vi "Close SV.vi"(8 "error in (no error)":errorcluster, 10 "Process Name":string="Flow Module 1", 11 "State Cluster in":T1={"Settings"={"Feed Module Configuration"={"Cycle Period"=0.0, "Ismatech"={"VISA resource name"="", "Simulated?"=FALSE, "Pump Number"=1.0, "Reverse?"=FALSE}, "Masterflex"={"VISA resource name"="", "Simulated?"=FALSE, "Pump Number"=1.0, "Reverse?"=FALSE}, "Mettler"={"VISA resource name"="", "Simulated?"=FALSE}, "Bronkhorst M13 Flow Meter"={"VISA resource name"="", "Simulated?"=FALSE, "Smoothing Steps"=1}, "PID 2 Parameters"={"Input Device"=enum."Flowmeter", "Output Device"=enum."Ismatec ISM 831C", "Setpoint"=0.0, "PID gains"={"proportional gain (Kc)"=1.0, "integral time (Ti, min)"=0.01, "derivative time (Td, min)"=0.0}}, "Manual Entry"=0.0, "Auto?"=TRUE, "VICI Settings"={"VISA resource name"="", "Simulated?"=FALSE, "Pump Number"=0.0, "Reverse?"=FALSE}, "output range"={"output high"=100.0, "output low"=0.0}}, "Load Count"=0.0, "TT Configuration In"={"physical channels"="cDAQ2Mod4/ai0", "name to assign"="Temp1", "units"=10143}, "PT Configuration"={"physical channels"="cDAQ2Mod8/ai15", "name to assign"="Pressure", "units"=10342}}, "Shared Variables"={"PID 1 Process Variable"="PID1-Mettler Toledo Scale 1", "PID 1 Output"="PID1-Mettler Toledo Scale 1", "PID 1 Setpoint"="PID1-Setpoint", "PID 1 Setpoint SV refnum"="ni.var.psp://localhost/Flow Module 1/PID1-Setpoint", "PID 1 Process Variable SV refnum"="ni.var.psp://localhost/Flow Module 1/PID1-Setpoint", "PID 1 Output SV refnum"="ni.var.psp://localhost/Flow Module 1/PID1-Setpoint"}, "Feed Module Config"={"GUID"="", "Drop Coords"={"Horizontal"=0, "Vertical"=0}, "Process Name"="", "Settings"={"Cycle Period"=500.0, "Ismatech"={"VISA resource name"="", "Simulated?"=TRUE, "Pump Number"=1.0, "Reverse?"=FALSE}, "Masterflex"={"VISA resource name"="", "Simulated?"=TRUE, "Pump Number"=1.0, "Reverse?"=FALSE}, "Mettler"={"VISA resource name"="", "Simulated?"=FALSE}, "Bronkhorst M13 Flow Meter"={"VISA resource name"="", "Simulated?"=TRUE, "Smoothing Steps"=1}, "PID 2 Parameters"={"Input Device"=enum."Default", "Output Device"=enum."Default", "Setpoint"=0.0, "PID gains"={"proportional gain (Kc)"=1.0, "integral time (Ti, min)"=0.01, "derivative time (Td, min)"=0.0}}, "Manual Entry"=0.0, "Auto?"=TRUE, "VICI Settings"={"VISA resource name"="", "Simulated?"=TRUE, "Pump Number"=0.0, "Reverse?"=FALSE}, "output range"={"output high"=100.0, "output low"=0.0}}, "Load Count"=0}} {"Feed Module Config"."Settings"."output range"."output low" min=0.0 max=100.0 format="%.2f"; "Feed Module Config"."Settings"."output range"."output high" format="%.2f"; "Feed Module Config"."Settings"."VICI Settings"."Pump Number" min=1.0 max=20.0 step=1.0; "Feed Module Config"."Settings"."PID 2 Parameters"."PID gains"."derivative time (Td, min)" format="%.3f"; "Feed Module Config"."Settings"."PID 2 Parameters"."PID gains"."integral time (Ti, min)" format="%.3f"; "Feed Module Config"."Settings"."PID 2 Parameters"."PID gains"."proportional gain (Kc)" format="%.3f"; "Feed Module Config"."Settings"."Bronkhorst M13 Flow Meter"."Smoothing Steps" min=1 step=1; "Feed Module Config"."Settings"."Masterflex"."Pump Number" min=1.0 max=20.0 step=1.0; "Feed Module Config"."Settings"."Ismatech"."Pump Number" min=1.0 max=20.0 step=1.0; "Settings"."PT Configuration"."units" items=["Amps"=10342, "From Custom Scale"=10065]; "Settings"."TT Configuration In"."units" items=["Deg C"=10143, "Deg F"=10144, "Kelvins"=10325, "Deg R"=10145, "From Custom Scale"=10065]; "Settings"."Feed Module Configuration"."output range"."output low" min=0.0 max=100.0 format="%.2f"; "Settings"."Feed Module Configuration"."output range"."output high" format="%.2f"; "Settings"."Feed Module Configuration"."VICI Settings"."Pump Number" min=1.0 max=20.0 step=1.0; "Settings"."Feed Module Configuration"."PID 2 Parameters"."PID gains"."derivative time (Td, min)" format="%.3f"; "Settings"."Feed Module Configuration"."PID 2 Parameters"."PID gains"."integral time (Ti, min)" format="%.3f"; "Settings"."Feed Module Configuration"."PID 2 Parameters"."PID gains"."proportional gain (Kc)" format="%.3f"; "Settings"."Feed Module Configuration"."Bronkhorst M13 Flow Meter"."Smoothing Steps" min=1 step=1; "Settings"."Feed Module Configuration"."Masterflex"."Pump Number" min=1.0 max=20.0 step=1.0; "Settings"."Feed Module Configuration"."Ismatech"."Pump Number" min=1.0 max=20.0 step=1.0}) -> (0 "error out":errorcluster, 3 "State Cluster out":T1={"Settings"={"Feed Module Configuration"={"Cycle Period"=0.0, "Ismatech"={"VISA resource name"="", "Simulated?"=FALSE, "Pump Number"=1.0, "Reverse?"=FALSE}, "Masterflex"={"VISA resource name"="", "Simulated?"=FALSE, "Pump Number"=1.0, "Reverse?"=FALSE}, "Mettler"={"VISA resource name"="", "Simulated?"=FALSE}, "Bronkhorst M13 Flow Meter"={"VISA resource name"="", "Simulated?"=FALSE, "Smoothing Steps"=1}, "PID 2 Parameters"={"Input Device"=enum."Flowmeter", "Output Device"=enum."Ismatec ISM 831C", "Setpoint"=0.0, "PID gains"={"proportional gain (Kc)"=1.0, "integral time (Ti, min)"=0.01, "derivative time (Td, min)"=0.0}}, "Manual Entry"=0.0, "Auto?"=TRUE, "VICI Settings"={"VISA resource name"="", "Simulated?"=FALSE, "Pump Number"=0.0, "Reverse?"=FALSE}, "output range"={"output high"=100.0, "output low"=0.0}}, "Load Count"=0.0, "TT Configuration In"={"physical channels"="cDAQ2Mod4/ai0", "name to assign"="Temp1", "units"=10143}, "PT Configuration"={"physical channels"="cDAQ2Mod8/ai15", "name to assign"="Pressure", "units"=10342}}, "Shared Variables"={"PID 1 Process Variable"="PID1-Mettler Toledo Scale 1", "PID 1 Output"="PID1-Mettler Toledo Scale 1", "PID 1 Setpoint"="PID1-Setpoint", "PID 1 Setpoint SV refnum"="ni.var.psp://localhost/Flow Module 1/PID1-Setpoint", "PID 1 Process Variable SV refnum"="ni.var.psp://localhost/Flow Module 1/PID1-Setpoint", "PID 1 Output SV refnum"="ni.var.psp://localhost/Flow Module 1/PID1-Setpoint"}, "Feed Module Config"={"GUID"="", "Drop Coords"={"Horizontal"=0, "Vertical"=0}, "Process Name"="", "Settings"={"Cycle Period"=500.0, "Ismatech"={"VISA resource name"="", "Simulated?"=TRUE, "Pump Number"=1.0, "Reverse?"=FALSE}, "Masterflex"={"VISA resource name"="", "Simulated?"=TRUE, "Pump Number"=1.0, "Reverse?"=FALSE}, "Mettler"={"VISA resource name"="", "Simulated?"=FALSE}, "Bronkhorst M13 Flow Meter"={"VISA resource name"="", "Simulated?"=TRUE, "Smoothing Steps"=1}, "PID 2 Parameters"={"Input Device"=enum."Default", "Output Device"=enum."Default", "Setpoint"=0.0, "PID gains"={"proportional gain (Kc)"=1.0, "integral time (Ti, min)"=0.01, "derivative time (Td, min)"=0.0}}, "Manual Entry"=0.0, "Auto?"=TRUE, "VICI Settings"={"VISA resource name"="", "Simulated?"=TRUE, "Pump Number"=0.0, "Reverse?"=FALSE}, "output range"={"output high"=100.0, "output low"=0.0}}, "Load Count"=0}} {"Feed Module Config"."Settings"."output range"."output low" min=0.0 max=100.0 format="%.2f"; "Feed Module Config"."Settings"."output range"."output high" format="%.2f"; "Feed Module Config"."Settings"."VICI Settings"."Pump Number" min=1.0 max=20.0 step=1.0; "Feed Module Config"."Settings"."PID 2 Parameters"."PID gains"."derivative time (Td, min)" format="%.3f"; "Feed Module Config"."Settings"."PID 2 Parameters"."PID gains"."integral time (Ti, min)" format="%.3f"; "Feed Module Config"."Settings"."PID 2 Parameters"."PID gains"."proportional gain (Kc)" format="%.3f"; "Feed Module Config"."Settings"."Bronkhorst M13 Flow Meter"."Smoothing Steps" min=1 step=1; "Feed Module Config"."Settings"."Masterflex"."Pump Number" min=1.0 max=20.0 step=1.0; "Feed Module Config"."Settings"."Ismatech"."Pump Number" min=1.0 max=20.0 step=1.0; "Settings"."PT Configuration"."units" items=["Amps"=10342, "From Custom Scale"=10065]; "Settings"."TT Configuration In"."units" items=["Deg C"=10143, "Deg F"=10144, "Kelvins"=10325, "Deg R"=10145, "From Custom Scale"=10065]; "Settings"."Feed Module Configuration"."output range"."output low" min=0.0 max=100.0 format="%.2f"; "Settings"."Feed Module Configuration"."output range"."output high" format="%.2f"; "Settings"."Feed Module Configuration"."VICI Settings"."Pump Number" min=1.0 max=20.0 step=1.0; "Settings"."Feed Module Configuration"."PID 2 Parameters"."PID gains"."derivative time (Td, min)" format="%.3f"; "Settings"."Feed Module Configuration"."PID 2 Parameters"."PID gains"."integral time (Ti, min)" format="%.3f"; "Settings"."Feed Module Configuration"."PID 2 Parameters"."PID gains"."proportional gain (Kc)" format="%.3f"; "Settings"."Feed Module Configuration"."Bronkhorst M13 Flow Meter"."Smoothing Steps" min=1 step=1; "Settings"."Feed Module Configuration"."Masterflex"."Pump Number" min=1.0 max=20.0 step=1.0; "Settings"."Feed Module Configuration"."Ismatech"."Pump Number" min=1.0 max=20.0 step=1.0})   [LabVIEW 2021, in "Scale Module.lvlib"]
uses:
  Scale Module.lvlib
  Shared Variables/Dynamic Shared Variables.lvlib
  Controls/Scale Module Shared Variable Cluster.ctl
  Controls/Scale Module Settings Cluster.ctl
  Settings/Settings.ctl
  Settings/Settings.lvlib
  Controls/Scale Module State Cluster.ctl
  Ismatec ISM 831C/Controls/Ismatech Settings Cluster.ctl
  Masterflex 7550-30/Controls/Settings Cluster.ctl
  Masterflex 7550-30/Masterflex 7550-30.lvlib
  Mettler Toledo/Controls/Settings Cluster.ctl
  Mettler Toledo/Mettler Toledo.lvlib
  Bronkhorst M13 Flow Meter/Settings Cluster.ctl
  Bronkhorst M13 Flow Meter/Bronkhorst M13 Flow Meter.lvlib
  Measure Instrument/PID Input Enum.ctl
  Measure Instrument/PID 2 Output Enum.ctl
  Measure Instrument/PID 2 Parameters Cluster.ctl
  Pressure Sensor/PT Configuration.ctl
  Pressure Sensor/Pressure.lvlib
  VICI M50/VICI Settings.ctl
  <vilib>/Utility/miscctls.llb/LVPoint32TypeDef.ctl
  Controls/Scale Module Config Cluster.ctl
panel:
  # "Output Instruments"
  # "Input Instruments"
  # "Output Instruments"
  # "Input Instruments"
  # "Output Instruments"
  # "Input Instruments"
  # "Output Instruments"
  # "Input Instruments"
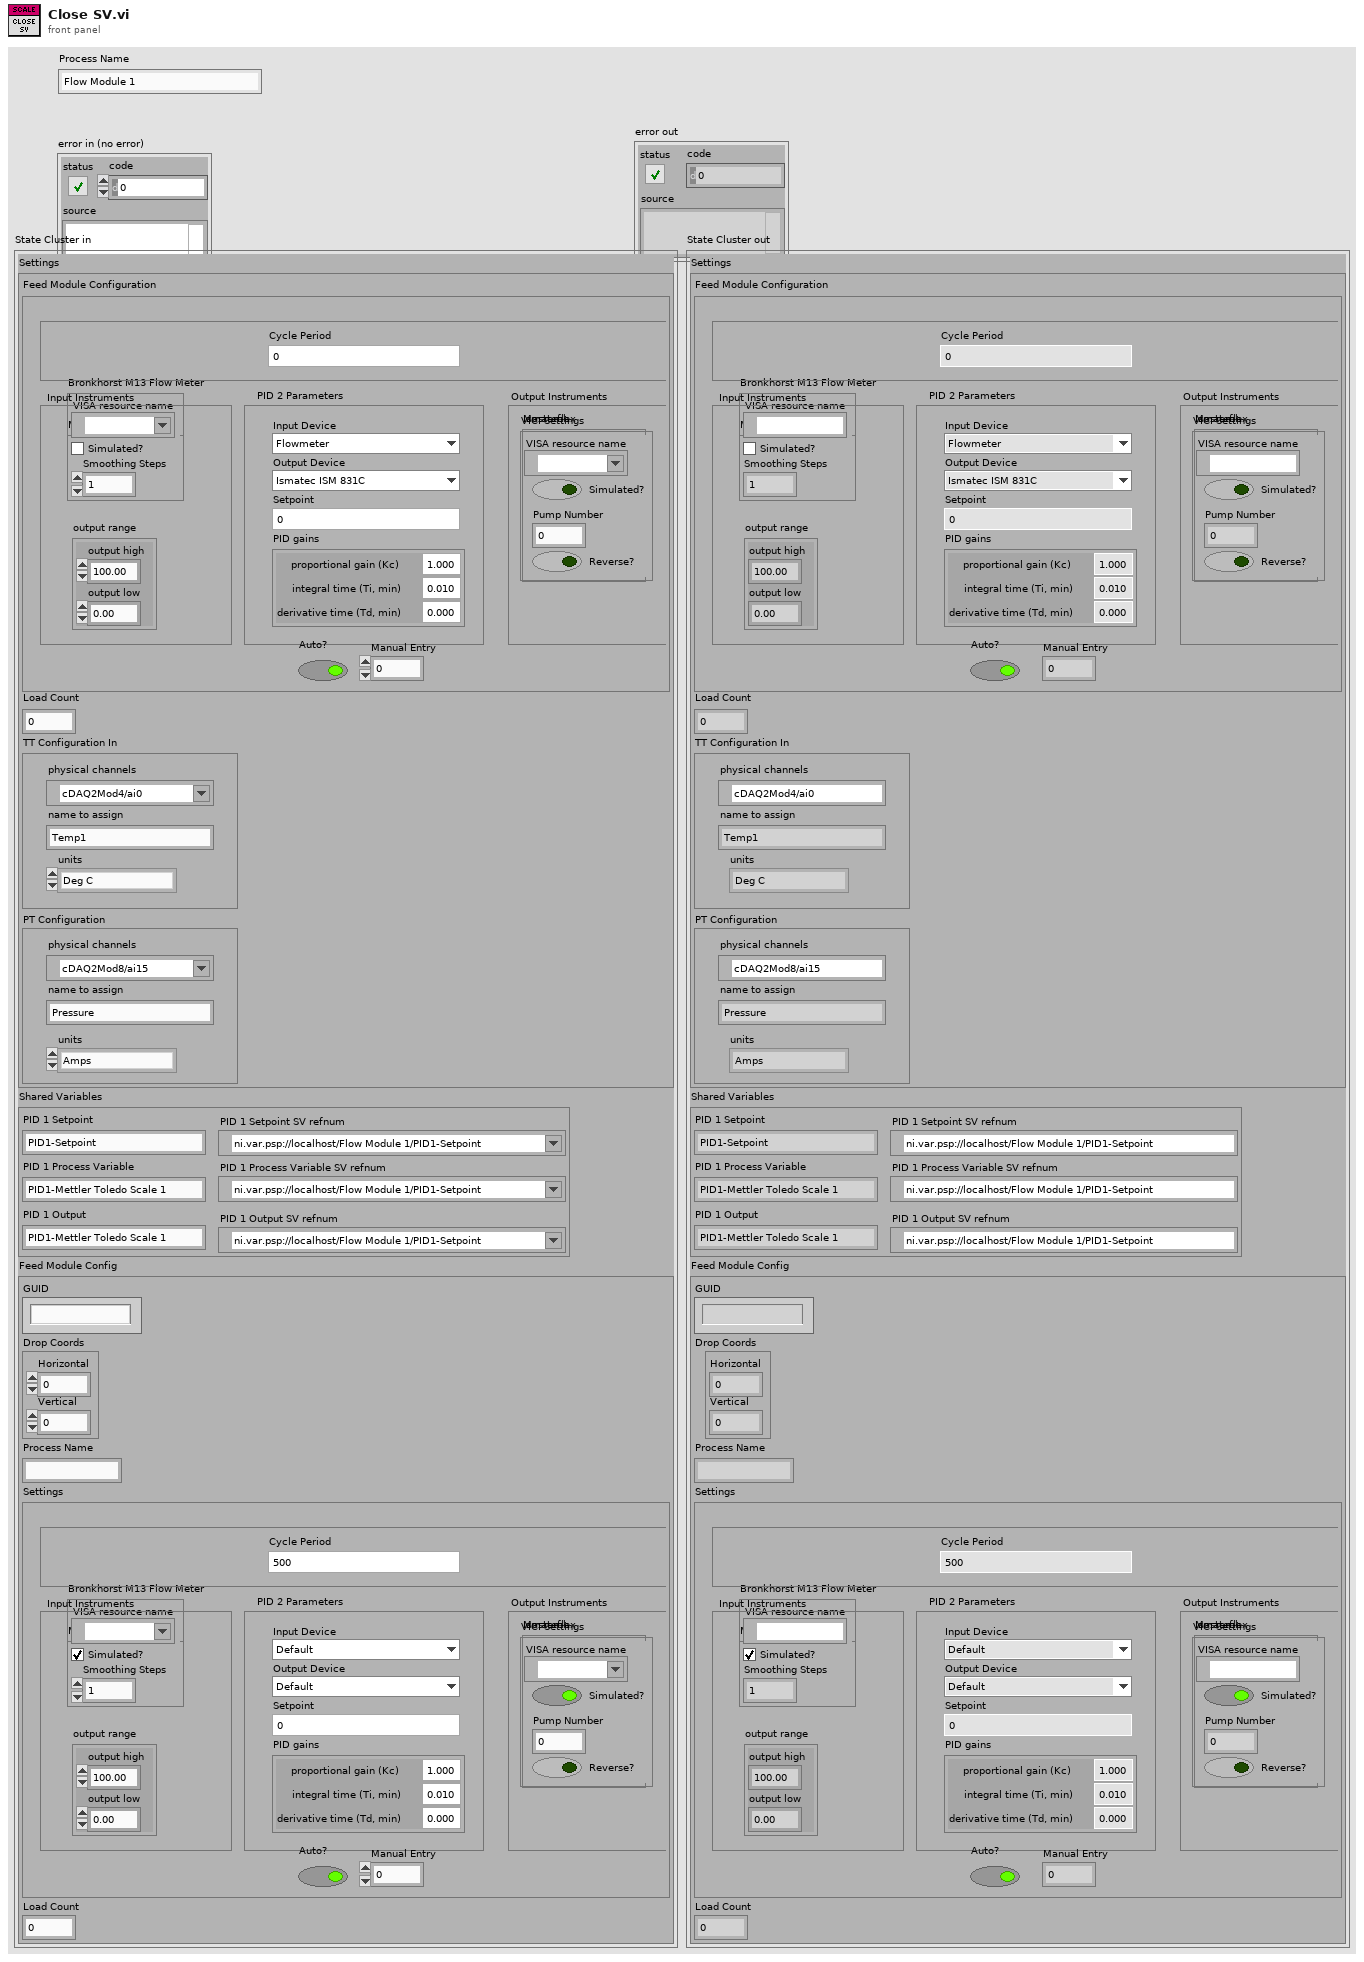
[diagram p1: front panel]
types:
  T1 = typedef "Scale Module.lvlib/Scale Module State Cluster.ctl" = cluster{"Settings":T2, "Shared Variables":T13, "Feed Module Config":T14}
  T2 = typedef "Settings.lvlib/Settings.ctl" = cluster{"Feed Module Configuration":T3, "Load Count":dbl, "TT Configuration In":cluster{"physical channels":tag, "name to assign":string, "units":i32}, "PT Configuration":T12}
  T3 = typedef "Scale Module.lvlib/Scale Module Settings Cluster.ctl" = cluster{"Cycle Period":dbl, "Ismatech":T4, "Masterflex":T5, "Mettler":T6, "Bronkhorst M13 Flow Meter":T7, "PID 2 Parameters":T8, "Manual Entry":dbl, "Auto?":bool, "VICI Settings":T11, "output range":cluster{"output high":dbl, "output low":dbl}}
  T4 = typedef "Ismatec ISM 831C.lvlib/Ismatech Settings Cluster.ctl" = cluster{"VISA resource name":refnum<visa-resource-name>, "Simulated?":bool, "Pump Number":dbl, "Reverse?":bool}
  T5 = typedef "Masterflex 7550-30.lvlib/Settings Cluster.ctl" = cluster{"VISA resource name":refnum<visa-resource-name>, "Simulated?":bool, "Pump Number":dbl, "Reverse?":bool}
  T6 = typedef "Mettler Toledo.lvlib/Settings Cluster.ctl" = cluster{"VISA resource name":refnum<visa-resource-name>, "Simulated?":bool}
  T7 = typedef "Bronkhorst M13 Flow Meter.lvlib/Settings Cluster.ctl" = cluster{"VISA resource name":refnum<visa-resource-name>, "Simulated?":bool, "Smoothing Steps":i32}
  T8 = typedef "PID 2 Parameters Cluster.ctl" = cluster{"Input Device":T9, "Output Device":T10, "Setpoint":dbl, "PID gains":cluster{"proportional gain (Kc)":dbl, "integral time (Ti, min)":dbl, "derivative time (Td, min)":dbl}}
  T9 = typedef "PID Input Enum.ctl" = enum16{"Default", "Flowmeter", "Scale Rate of Change"}
  T10 = typedef "PID 2 Output Enum.ctl" = enum16{"Default", "Ismatec ISM 4308", "Ismatec ISM 831C", "Masterflex 7550-30", "VICI M6", "VICI M50", "Tacmina QI", "KNF SIMDOS", "ASIA Type C", "FLOM UI-22-11", "SSI PR/LD", "SSI P40", "Masterflex 75211-70"}
  T11 = typedef "VICI Settings.ctl" = cluster{"VISA resource name":refnum<visa-resource-name>, "Simulated?":bool, "Pump Number":dbl, "Reverse?":bool}
  T12 = typedef "Pressure.lvlib/PT Configuration.ctl" = cluster{"physical channels":tag, "name to assign":string, "units":i32}
  T13 = typedef "Scale Module.lvlib/Scale Module Shared Variable Cluster.ctl" = cluster{"PID 1 Process Variable":string, "PID 1 Output":string, "PID 1 Setpoint":string, "PID 1 Setpoint SV refnum":refnum<k21>, "PID 1 Process Variable SV refnum":refnum<k21>, "PID 1 Output SV refnum":refnum<k21>}
  T14 = typedef "Scale Module.lvlib/Scale Module Config Cluster.ctl" = cluster{"GUID":string, "Drop Coords":T15, "Process Name":string, "Settings":T16, "Load Count":i32}
  T15 = typedef "LVPoint32TypeDef.ctl" = cluster{"Horizontal":i32, "Vertical":i32}
  T16 = typedef "Scale Module.lvlib/Scale Module Settings Cluster.ctl" = cluster{"Cycle Period":dbl, "Ismatech":T4, "Masterflex":T5, "Mettler":T6, "Bronkhorst M13 Flow Meter":T7, "PID 2 Parameters":T17, "Manual Entry":dbl, "Auto?":bool, "VICI Settings":T11, "output range":cluster{"output high":dbl, "output low":dbl}}
  T17 = typedef "PID 2 Parameters Cluster.ctl" = cluster{"Input Device":T18, "Output Device":T10, "Setpoint":dbl, "PID gains":cluster{"proportional gain (Kc)":dbl, "integral time (Ti, min)":dbl, "derivative time (Td, min)":dbl}}
  T18 = typedef "PID Input Enum.ctl" = enum16{"Default", "Bronkhorst M13", "Bronkhorst M14", "Scale Rate of Change"}
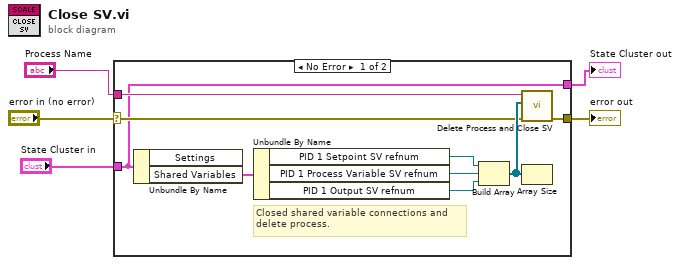
[diagram p0: block diagram]
diagram:
  n1 = case shown="No Error" "error in (no error)" {
    selector: "error in (no error)" -> [w8 w16]
    tunnel: "Process Name" -> [w13 _]
    tunnel: [w7 w16] -> w3
    tunnel: "State Cluster in" -> [w6 w15]
    tunnel: [w6 w15] -> w1
    frame No Error {
      # "Closed shared variable connections and\ndelete process."
      n2 = Unbundle By Name(w6) -> ("Shared Variables"=w14:T13)  [unwired: 1 out]
      n3 = Unbundle By Name(w14) -> ("PID 1 Setpoint SV refnum"=w12:refnum<k21>, "PID 1 Process Variable SV refnum"=w11:refnum<k21>, "PID 1 Output SV refnum"=w10:refnum<k21>)
      n4 = Build Array(w12, w11, w10) -> (w9:refnum<k21>[])
      n5 = call "Delete Process and Close SV.vi"("error in (no error)"=w8, "Array"=w9, "process name"=w13) -> ("error out"=w7:errorcluster)  [unwired: 8 in]
      n6 = Array Size(array=w9) -> ()  [unwired: 1 out]
    }
    frame Error {
    }
  }
  "error out" <- w3
  "State Cluster out" <- w1
